vi "GetLowPrioritySensors.vi"() -> ()   [LabVIEW 2020]
doc: "All low priority sensor reads should be placed in this VI."
uses:
  refnums.vi
  GRNF_Compressor.vi
  sensors.vi
  GRNF_CTREMotor.vi
  <vilib>/Rock Robotics/WPI/ThirdParty/Phoenix-LabVIEW/Motor Controller/Get/CTRE_Phoenix_MotorController_GetTemperature.vi
  robotprofile.vi
panel:
  out "Pressure Change (psi/min)":dbl
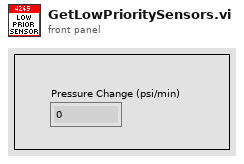
[diagram p1: front panel]
types:
  T1 = typedef "WPI_MotorControlDeviceRef.ctl" = cluster{"DeviceStatus":errorcluster, "Type":T2, "PWM":cluster{"PWM Channel":T3, "DeadBand":T4}, "CAN":cluster{"Device Number":u8, "SetOutput VI Ref":variant, "GetOutput VI Ref":variant, "Enable VI Ref":variant, "Disable VI Ref":variant, "Data":variant}, "Invert":bool, "DIO PWM":cluster{"PWM \"Enable\" Channel":T3, "DIOChannel":T5, "PWM Rate":dbl}}
  T2 = typedef "WPI_MotorControlType.ctl" = enum16{"PWM", "CAN", "DIO PWM"}
  T3 = typedef "FPGA_DIOPWMChannel.ctl" = enum8{"PWM 0", "PWM 1", "PWM 2", "PWM 3", "PWM 4", "PWM 5", "PWM 6", "PWM 7", "PWM 8", "PWM 9", "PWM MXP 0", "PWM MXP 1", "PWM MXP 2", "PWM MXP 3", "PWM MXP 4", "PWM MXP 5", "PWM MXP 6", "PWM MXP 7", "PWM MXP 8", "PWM MXP 9", "Invalid"}
  T4 = typedef "WPI_PWMDeadband.ctl" = cluster{"Name":string, "maxPositivePwm":i32, "minPositivePwm":i32, "centerPwm":i32, "maxNegativePwm":i32, "minNegativePwm":i32, "angularRange":u16}
  T5 = typedef "FPGA_DIOChannel.ctl" = enum8{"DIO 0", "DIO 1", "DIO 2", "DIO 3", "DIO 4", "DIO 5", "DIO 6", "DIO 7", "DIO 8", "DIO 9", "DIO MXP 0", "DIO MXP 1", "DIO MXP 2", "DIO MXP 3", "DIO MXP 4", "DIO MXP 5", "DIO MXP 6", "DIO MXP 7", "DIO MXP 8", "DIO MXP 9", "DIO MXP 10", "DIO MXP 11", "DIO MXP 12", "DIO MXP 13", "DIO MXP 14", "DIO MXP 15", "SPI Port CS1", "SPI Port CS2", "SPI Port CS3", "SPI Port MISO", "SPI Port MOSI", "Invalid"}
  T6 = typedef "WPI_CompressorDevRef.ctl" = cluster{"DevStatus":errorcluster, "Pneumatics Control Module":u8}
  T7 = cluster{"Battery Voltage Fault":bool, "Hardware Fault":bool, "CAN Warning Fault":bool, "Temperature Fault":bool}
  T8 = cluster{"HardwareFault":bool, "CompressorFault":bool, "SolenoidFault":bool, "Compressor Open":bool, "Brownout":bool}
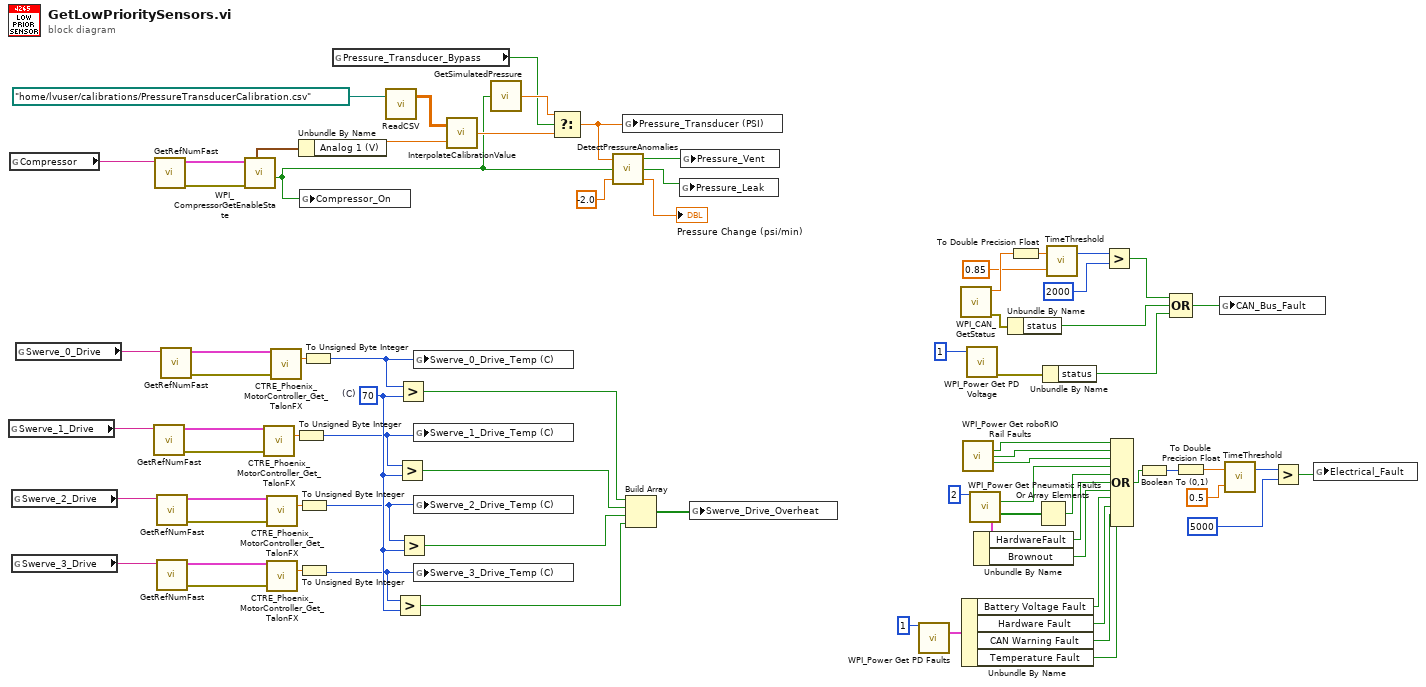
[diagram p0: block diagram]
diagram:
  w74 = u8 70  # (C)
  n1 = global read "refnums.vi" "Swerve_1_Drive"() -> (w62:string)
  n2 = global read "refnums.vi" "Compressor"() -> (w75:string)
  n3 = global read "refnums.vi" "Swerve_2_Drive"() -> (w58:string)
  n4 = global read "refnums.vi" "Swerve_3_Drive"() -> (w54:string)
  n5 = global read "refnums.vi" "Swerve_0_Drive"() -> (w68:string)
  n6 = call-poly "GetRefNumFast.vi"("RefNum Name"=w62) -> ("Error"=w60:errorcluster, "Device Reference"=w61:T1)  [unwired: 5 in]
  n7 = call-poly "GetRefNumFast.vi"("RefNum Name"=w75) -> ("Error"=w21:errorcluster, "Device Reference"=w22:T6)  [unwired: 5 in]
  n8 = call-poly "GetRefNumFast.vi"("RefNum Name"=w58) -> ("Error"=w56:errorcluster, "Device Reference"=w57:T1)  [unwired: 5 in]
  n9 = call-poly "GetRefNumFast.vi"("RefNum Name"=w54) -> ("Error"=w52:errorcluster, "Device Reference"=w53:T1)  [unwired: 5 in]
  n10 = call-poly "GetRefNumFast.vi"("RefNum Name"=w68) -> ("Error"=w65:errorcluster, "Device Reference"=w66:T1)  [unwired: 5 in]
  n11 = call <vilib>:"WPI_CompressorGetEnableState.vi"("error in (no error)"=w21, "CompressorDevRef"=w22) -> ("Compressor Running"=w20:bool, "Analog  Sensors"=w19:cluster{"Analog 0 (V)":dbl, "Analog 1 (V)":dbl})  [unwired: 3 in, 5 out]
  n12 = call-poly <vilib>:"CTRE_Phoenix_MotorController_Get_TalonFX.vi"("PhoenixMotorControlDevRef"=w61, "error in"=w60) -> ("Temperature (C)"=w59:dbl)  [unwired: 11 in, 2 out]
  n13 = call-poly <vilib>:"CTRE_Phoenix_MotorController_Get_TalonFX.vi"("PhoenixMotorControlDevRef"=w57, "error in"=w56) -> ("Temperature (C)"=w55:dbl)  [unwired: 11 in, 2 out]
  n14 = call-poly <vilib>:"CTRE_Phoenix_MotorController_Get_TalonFX.vi"("PhoenixMotorControlDevRef"=w53, "error in"=w52) -> ("Temperature (C)"=w51:dbl)  [unwired: 11 in, 2 out]
  n15 = call-poly <vilib>:"CTRE_Phoenix_MotorController_Get_TalonFX.vi"("PhoenixMotorControlDevRef"=w66, "error in"=w65) -> ("Temperature (C)"=w64:dbl)  [unwired: 11 in, 2 out]
  n16 = To Unsigned Byte Integer(number=w59) -> (unsigned 8bit integer=w48:u8)
  n17 = Unbundle By Name(w19) -> ("Analog 1 (V)"=w18:dbl)
  n18 = To Unsigned Byte Integer(number=w55) -> (unsigned 8bit integer=w50:u8)
  n19 = To Unsigned Byte Integer(number=w51) -> (unsigned 8bit integer=w49:u8)
  n20 = global write "sensors.vi" "Compressor_On"(w20) -> ()
  n21 = To Unsigned Byte Integer(number=w64) -> (unsigned 8bit integer=w63:u8)
  n22 = global read "robotprofile.vi" "Pressure_Transducer_Bypass"() -> (w28:bool)
  n23 = call "ReadCSV.vi"("File Path (.csv)"=path "/home/lvuser/calibrations/PressureTransducerCalibration.csv" ("path")) -> ("Data (index by row)"=w76:dbl[][])  [unwired: 1 in, 1 out]
  n24 = Greater?(x=w49, y=w74) -> (0:w70:bool)
  n25 = Greater?(x=w48, y=w74) -> (0:w72:bool)
  n26 = Greater?(x=w63, y=w74) -> (0:w73:bool)
  n27 = Greater?(x=w50, y=w74) -> (0:w71:bool)
  n28 = global write "sensors.vi" "Swerve_0_Drive_Temp (C)"(w63) -> ()
  n29 = global write "sensors.vi" "Swerve_1_Drive_Temp (C)"(w48) -> ()
  n30 = global write "sensors.vi" "Swerve_2_Drive_Temp (C)"(w50) -> ()
  n31 = global write "sensors.vi" "Swerve_3_Drive_Temp (C)"(w49) -> ()
  n32 = call "InterpolateCalibrationValue.vi"("Input"=w18, "Calibration Data"=w76) -> ("Interpolated Output"=w29:dbl)
  n33 = call "GetSimulatedPressure.vi"("Compressor On"=w20) -> ("Simulated Pressure Transducer"=w30:dbl)
  n34 = Select(t=w30, s=w28, f=w29) -> (s? t:f=w24:dbl)
  n35 = call "DetectPressureAnomalies.vi"("Pressure Loss Threshold (psi/min)"=-2.0, "Compressor Running"=w20, "Pressure (psi)"=w24) -> ("Pressure Change (psi/min)"=→"Pressure Change (psi/min)":dbl, "Pressure Leak"=w27:bool, "Pressure Vent"=w26:bool)
  n36 = global write "sensors.vi" "Pressure_Transducer (PSI)"(w24) -> ()
  n37 = Build Array(w73, w72, w71, w70) -> (w69:bool[])
  n38 = global write "sensors.vi" "Pressure_Leak"(w27) -> ()
  n39 = global write "sensors.vi" "Pressure_Vent"(w26) -> ()
  n40 = global write "sensors.vi" "Swerve_Drive_Overheat"(w69) -> ()
  n41 = call <vilib>:"WPI_Power Get PD Faults.vi"("Power Distribution (def)"=u8 1) -> ("Faults"=w11:T7)  [unwired: 11 in, 3 out]
  n42 = call <vilib>:"WPI_CAN_GetStatus.vi"() -> ("error out"=w47:errorcluster, "Percent Bus Utilization"=w43:sgl)  [unwired: 6 in, 4 out]
  n43 = Unbundle By Name(w11) -> ("Battery Voltage Fault"=w4:bool, "Hardware Fault"=w3:bool, "CAN Warning Fault"=w2:bool, "Temperature Fault"=w1:bool)
  n44 = call <vilib>:"WPI_Power Get roboRIO Rail Faults.vi"() -> ("3.3V User Rail Short"=w14:bool, "5 V User Rail Short"=w13:bool, "6 V User Rail Short"=w12:bool)  [unwired: 10 in, 3 out]
  n45 = call <vilib>:"WPI_Power Get PD Voltage.vi"("Power Distribution Panel (def)"=u8 1 ("Power Distribution Panel (0)")) -> ("error out"=w9:errorcluster)  [unwired: 13 in, 1 out]
  n46 = call <vilib>:"WPI_Power Get Pneumatic Faults.vi"("Pneumatics device (def)"=u8 2) -> ("Compressor Fault"=w16:bool, "All Solenoid Faults"=w15:bool[], "Faults"=w7:T8)  [unwired: 9 in, 3 out]
  n47 = Unbundle By Name(w7) -> ("HardwareFault"=w6:bool, "Brownout"=w5:bool)
  n48 = Unbundle By Name(w47) -> ("status"=w46:bool)
  n49 = To Double Precision Float(number=w43) -> (double precision float=w41:dbl)
  n50 = Or Array Elements(Boolean array=w15) -> (logical OR=w67:bool)
  n51 = Unbundle By Name(w9) -> ("status"=w44:bool)
  n52 = call "TimeThreshold.vi"("Threshold"=0.85, "Current Value"=w41) -> ("Time Above Threshold (ms)"=w40:u32)  [unwired: 1 out]
  n53 = Greater?(x=w40, y=u32 2000) -> (0:w38:bool)
  n54 = Compound Arithmetic op=OR(w14, w13, w12, w16, w67, w6, w5, w4, w3, w2, w1) -> (w37:bool)
  n55 = Boolean To (0,1)(Boolean=w37) -> (0, 1=w36:i16)
  n56 = Compound Arithmetic op=OR(w38, w46, w44) -> (w45:bool)
  n57 = To Double Precision Float(number=w36) -> (double precision float=w35:dbl)
  n58 = global write "sensors.vi" "CAN_Bus_Fault"(w45) -> ()
  n59 = call "TimeThreshold.vi"("Threshold"=0.5, "Current Value"=w35) -> ("Time Above Threshold (ms)"=w33:u32)  [unwired: 1 out]
  n60 = Greater?(x=w33, y=u32 5000) -> (0:w31:bool)
  n61 = global write "sensors.vi" "Electrical_Fault"(w31) -> ()
